vi "Get DATA.vi"(8 "error in (no error)":errorcluster, 11 "CAN Message in":refnum<class "CAN Message.lvclass">) -> (0 "error out":errorcluster, 2 "DATA":u8[](array[numeric]), 3 "CAN Message out":refnum<class "CAN Message.lvclass">)   [LabVIEW 2024, in "PCAN.lvlib" / "CAN Message.lvclass"]
uses:
  CAN Message.lvclass
  CAN Message.lvclass/CAN Message.ctl
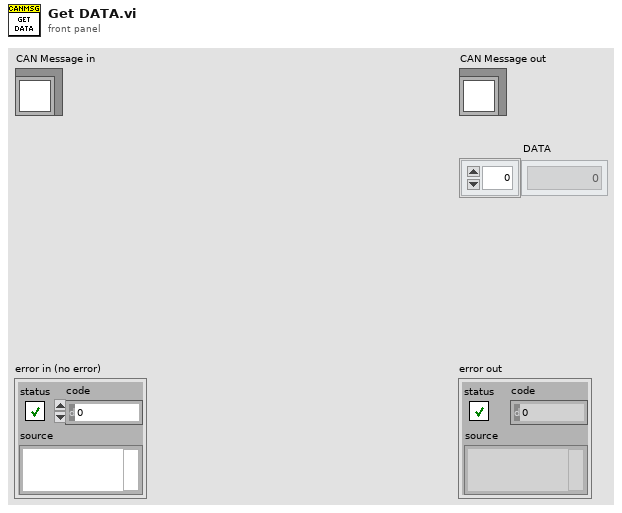
[diagram p1: front panel]
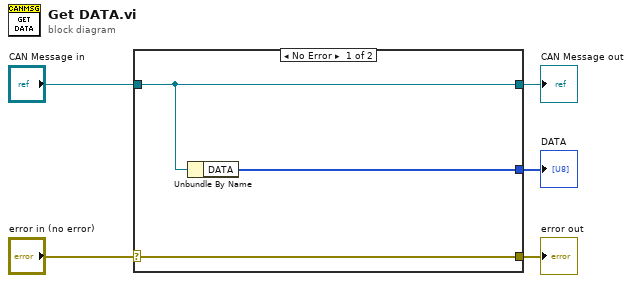
[diagram p0: block diagram]
diagram:
  n1 = case shown="No Error" "error in (no error)" {
    selector: "error in (no error)" -> [w8 w9]
    tunnel: [w8 w9] -> w4
    tunnel: [w7 w10] -> w2
    tunnel: "CAN Message in" -> [w7 w10]
    tunnel: [w6 _] -> w1
    frame No Error {
      n2 = Unbundle By Name(w7) -> ("DATA"=w6:u8[])
    }
    frame Error {
    }
  }
  "error out" <- w4
  "CAN Message out" <- w2
  "DATA" <- w1
